vi "Index Tags.vi"(4 "Write?":bool, 6 "Data Type":T1, 8 "error in (no error)":errorcluster, 9 "Tag":string, 10 "Group Index":i32, 11 "bt_Blackboard in":refnum<class "Blackboard.lvclass">) -> (0 "error out":errorcluster, 1 "New Tag?":bool, 2 "Index":i32, 3 "bt_Blackboard out":refnum<class "Blackboard.lvclass">)   [LabVIEW 2021, in "Blackboard.lvclass"]
uses:
  Blackboard.lvclass
  Data Type.ctl
  Blackboard.lvclass/Blackboard.ctl
  Status Type.ctl
  <vilib>/Utility/error.llb/Error Cluster From Error Code.vi
  <vilib>/ErrorRing/Error Ring.xnode
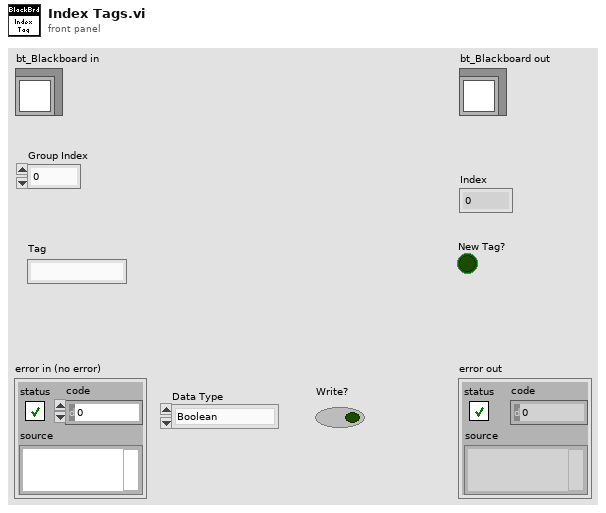
[diagram p1: front panel]
types:
  T1 = typedef "Blackboard.lvclass/Data Type.ctl" = enum16{"Boolean", "String", "DBL", "SGL", "EXT", "U8", "U16", "U32", "U64", "I8", "I16", "I32", "I64", "CDBL", "CSGL", "CEXT", "Time", "Variant", "Waveform"}
  T2 = typedef "Blackboard.lvclass/Status Type.ctl" = cluster{"Read?":u32, "Write?":u32, "Data Type":T1}
  T3 = typedef "Blackboard.lvclass/Data DVR Type.ctl" = cluster{"Tags":T4, "Status":refnum<data-value>, "Boolean":refnum<data-value>, "String":refnum<data-value>, "DBL":refnum<data-value>, "SGL":refnum<data-value>, "EXT":refnum<data-value>, "U8":refnum<data-value>, "U16":refnum<data-value>, "U32":refnum<data-value>, "U64":refnum<data-value>, "I8":refnum<data-value>, "I16":refnum<data-value>, "I32":refnum<data-value>, "I64":refnum<data-value>, "CDBL":refnum<data-value>, "CSGL":refnum<data-value>, "CEXT":refnum<data-value>, "Time":refnum<data-value>, "Variant":refnum<data-value>, "Waveform":refnum<data-value>}
  T4 = typedef "Blackboard.lvclass/Tags Map Type.ctl" = map{string, cluster{"Data Index":i32, "Status Index":i32}}
  T5 = typedef "Blackboard.lvclass/Group Map Type.ctl" = map{string, i32}
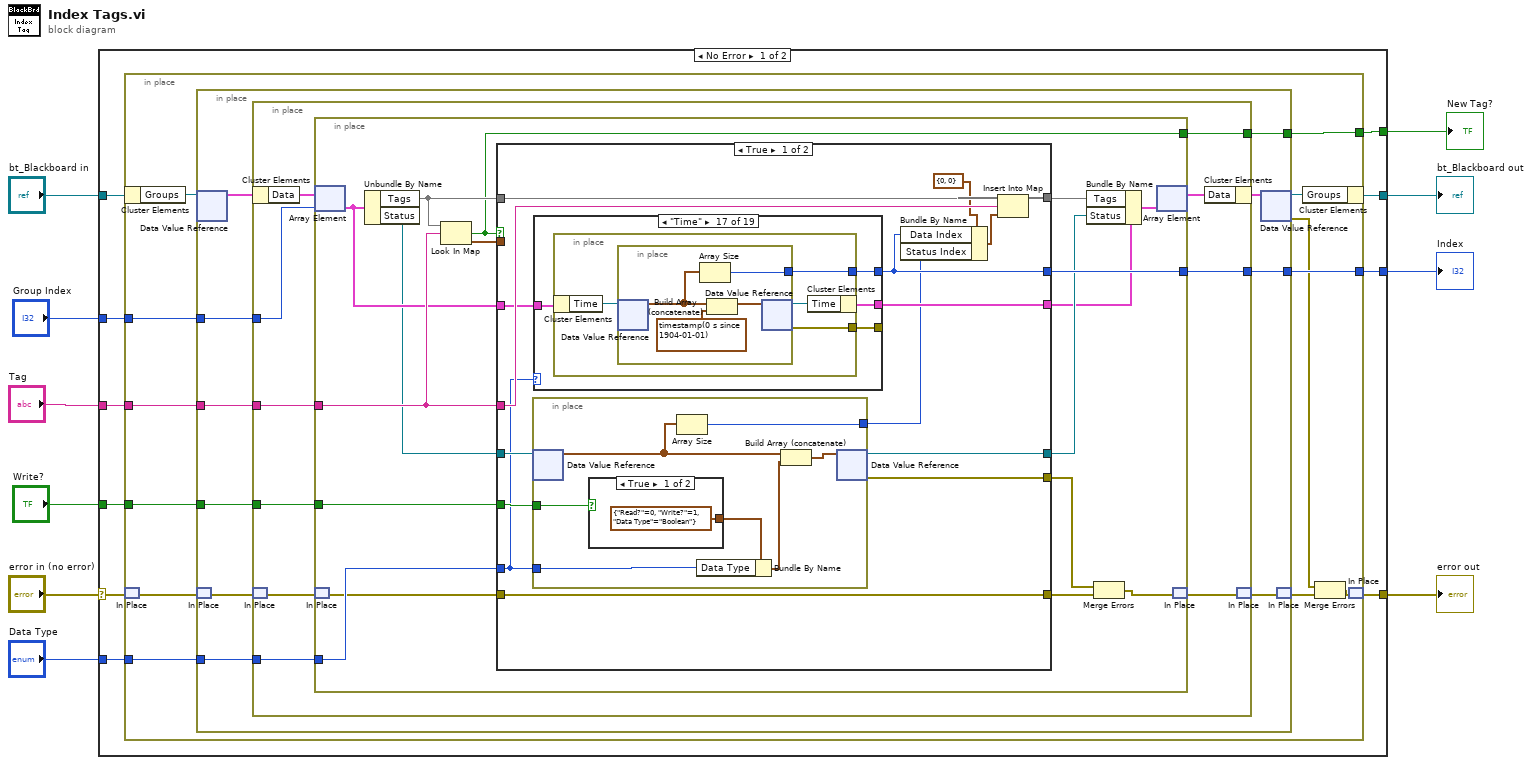
[diagram p0: block diagram]
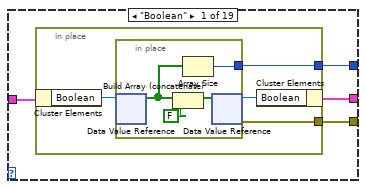
[diagram p2: hidden frame]
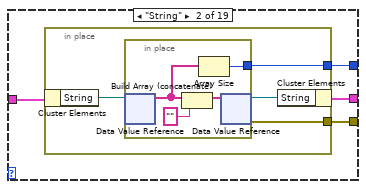
[diagram p3: hidden frame]
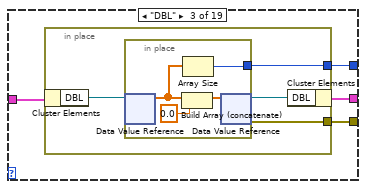
[diagram p4: hidden frame]
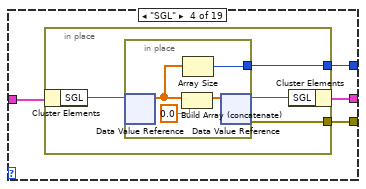
[diagram p5: hidden frame]
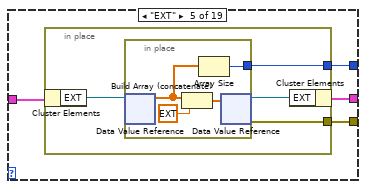
[diagram p6: hidden frame]
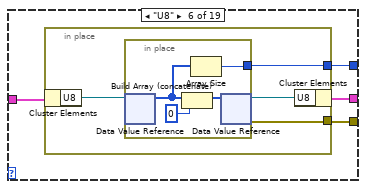
[diagram p7: hidden frame]
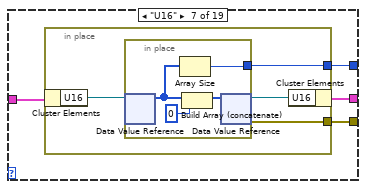
[diagram p8: hidden frame]
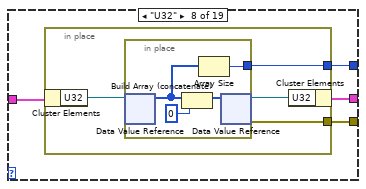
[diagram p9: hidden frame]
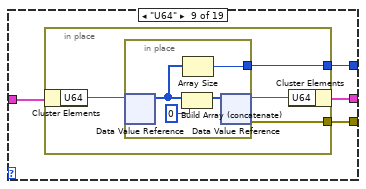
[diagram p10: hidden frame]
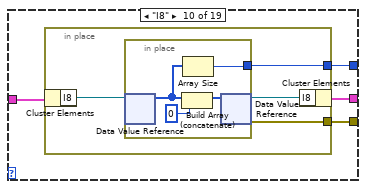
[diagram p11: hidden frame]
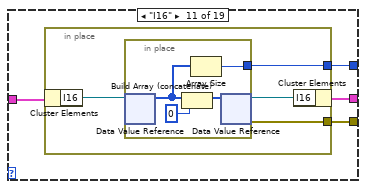
[diagram p12: hidden frame]
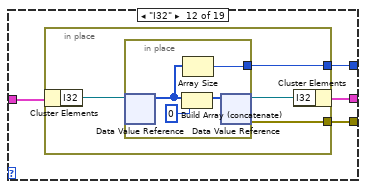
[diagram p13: hidden frame]
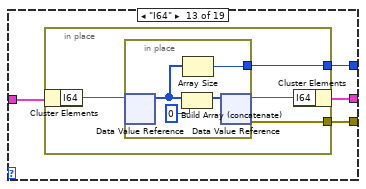
[diagram p14: hidden frame]
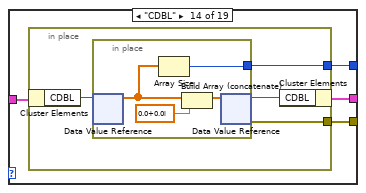
[diagram p15: hidden frame]
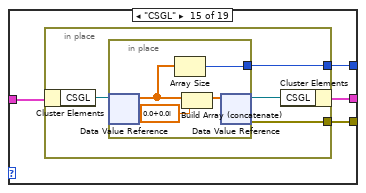
[diagram p16: hidden frame]
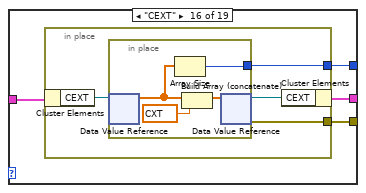
[diagram p17: hidden frame]
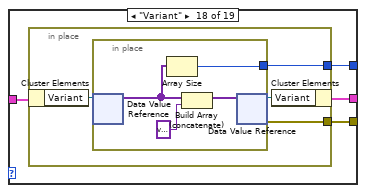
[diagram p18: hidden frame]
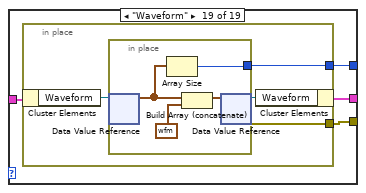
[diagram p19: hidden frame]
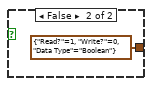
[diagram p20: hidden frame]
diagram:
  n1 = case shown="No Error" "error in (no error)" {
    selector: "error in (no error)" -> [w13 w366]
    tunnel: [w12 w366] -> w9
    tunnel: [w17 w365] -> w7
    tunnel: "bt_Blackboard in" -> [w18 w365]
    tunnel: "Tag" -> [w20 _]
    tunnel: [w19 _] -> w5
    tunnel: "Group Index" -> [w16 _]
    tunnel: "Write?" -> [w15 _]
    tunnel: "Data Type" -> [w14 _]
    tunnel: [w11 _] -> w1
    frame No Error {
      n2 = in-place {
        in-place-border: w20 -> [w32]
        in-place-border: [w31] -> w19
        in-place-border: w16 -> [w30]
        in-place-border: w15 -> [w29]
        in-place-border: w14 -> [w28]
        in-place-border: [w27] -> w11
        n3 = in-place-cluster #1(w18) -> ("Groups"=w26:refnum<data-value>)
        n4 = in-place-match #2(w13) -> (w25:errorcluster)
        n5 = in-place {
          in-place-border: w32 -> [w42]
          in-place-border: [w41] -> w31
          in-place-border: w30 -> [w40]
          in-place-border: w29 -> [w39]
          in-place-border: w28 -> [w38]
          in-place-border: [w37] -> w27
          n6 = in-place-dvr #3(w26) -> (w36:cluster{"Data":T3[], "Map":T5, "Status":u32[]})  [unwired: 1 out]
          n7 = in-place-match #4(w25) -> (w34:errorcluster)
          n8 = in-place {
            in-place-border: w42 -> [w52]
            in-place-border: [w51] -> w41
            in-place-border: w40 -> [w50]
            in-place-border: w39 -> [w49]
            in-place-border: w38 -> [w48]
            in-place-border: [w47] -> w37
            n9 = in-place-cluster #5(w36) -> ("Data"=w46:T3[])
            n10 = in-place-match #6(w34) -> (w44:errorcluster)
            n11 = in-place {
              in-place-border: w52 -> [w69]
              in-place-border: [w63] -> w51
              in-place-border: w49 -> [w68]
              in-place-border: w48 -> [w66]
              in-place-border: [w53] -> w47
              n12 = in-place-array #7(w46, w50) -> (w62:T3)
              n13 = in-place-match #8(w44) -> (w65:errorcluster)
              n14 = Unbundle By Name(w62) -> ("Tags"=w60:T4, "Status"=w57:refnum<data-value>)
              n15 = Look In Map(map=w60, key=w69) -> (key not found?=w53:bool, value=w58:cluster{"Data Index":i32, "Status Index":i32})  [unwired: 1 in]
              n16 = case shown="True" w53 {
                tunnel: w60 -> [w79 w327]
                tunnel: [w78 w327] -> w59
                tunnel: w69 -> [w77 _]
                tunnel: [w81 w324] -> w56
                tunnel: w68 -> [w84 w333]
                tunnel: w66 -> [w74 w332]
                tunnel: w65 -> [w83 w331]
                tunnel: [w83 w330] -> w61
                tunnel: w58 -> [_ w329]
                tunnel: [w73 w328] -> w63
                tunnel: w57 -> [w82 w325]
                tunnel: [w80 w323] -> w55
                tunnel: w62 -> [w76 w322]
                tunnel: [w75 w322] -> w54
                frame True {
                  n17 = in-place {
                    in-place-border: w84 -> [w319]
                    in-place-border: w74 -> [w315]
                    in-place-border: [w313] -> w70
                    n18 = in-place-dvr #9(w82) -> (w314:T2[])  [unwired: 1 out]
                    n19 = case shown="True" w319 {
                      tunnel: [T2 {"Read?"=0, "Write?"=1, "Data Type"=enum."Boolean"} ("Status") T2 {"Read?"=1, "Write?"=0, "Data Type"=enum."Boolean"} ("Status")] -> w318
                      frame True {
                      }
                      frame False {
                      }
                    }
                    n20 = Array Size(array=w314) -> (size(s)=w313:i32)
                    n21 = Bundle By Name(cluster=w318, "Data Type"=w315) -> (w316:T2)
                    n22 = Build Array (concatenate)(w314, w316) -> (w317:T2[])
                    n23 = in-place-dvr #9(w317) -> (w81:refnum<data-value>, w80:errorcluster)
                  }
                  n24 = case shown="\"Time\"" w74 {
                    tunnel: w76 -> [w88 w100 w112 w124 w136 w148 w160 w172 w184 w196 w208 w220 w232 w244 w256 w268 w280 w292 w304]
                    tunnel: [w87 w99 w111 w123 w135 w147 w159 w171 w183 w195 w207 w219 w231 w243 w255 w267 w279 w291 w303] -> w75
                    tunnel: [w86 w98 w110 w122 w134 w146 w158 w170 w182 w194 w206 w218 w230 w242 w254 w266 w278 w290 w302] -> _
                    tunnel: [w85 w97 w109 w121 w133 w145 w157 w169 w181 w193 w205 w217 w229 w241 w253 w265 w277 w289 w301] -> w73
                    frame "Boolean" {
                      n25 = in-place {
                        in-place-border: [w90] -> w86
                        in-place-border: [w89] -> w85
                        n26 = in-place-cluster #10(w88) -> ("Boolean"=w92:refnum<data-value>)
                        n27 = in-place {
                          in-place-border: [w93] -> w89
                          n28 = in-place-dvr #11(w92) -> (w94:bool[])  [unwired: 1 out]
                          n29 = Build Array (concatenate)(w94, FALSE) -> (w96:bool[])
                          n30 = Array Size(array=w94) -> (size(s)=w93:i32)
                          n31 = in-place-dvr #11(w96) -> (w91:refnum<data-value>, w90:errorcluster)
                        }
                        n32 = in-place-cluster #10("Boolean"=w91) -> (w87:T3)
                      }
                    }
                    frame "String" {
                      n33 = in-place {
                        in-place-border: [w102] -> w98
                        in-place-border: [w101] -> w97
                        n34 = in-place-cluster #12(w100) -> ("String"=w104:refnum<data-value>)
                        n35 = in-place {
                          in-place-border: [w105] -> w101
                          n36 = in-place-dvr #13(w104) -> (w106:string[])  [unwired: 1 out]
                          n37 = Build Array (concatenate)(w106, "") -> (w108:string[])
                          n38 = Array Size(array=w106) -> (size(s)=w105:i32)
                          n39 = in-place-dvr #13(w108) -> (w103:refnum<data-value>, w102:errorcluster)
                        }
                        n40 = in-place-cluster #12("String"=w103) -> (w99:T3)
                      }
                    }
                    frame "DBL" {
                      n41 = in-place {
                        in-place-border: [w114] -> w110
                        in-place-border: [w113] -> w109
                        n42 = in-place-cluster #14(w112) -> ("DBL"=w116:refnum<data-value>)
                        n43 = in-place {
                          in-place-border: [w117] -> w113
                          n44 = in-place-dvr #15(w116) -> (w118:dbl[])  [unwired: 1 out]
                          n45 = Build Array (concatenate)(w118, 0.0) -> (w120:dbl[])
                          n46 = Array Size(array=w118) -> (size(s)=w117:i32)
                          n47 = in-place-dvr #15(w120) -> (w115:refnum<data-value>, w114:errorcluster)
                        }
                        n48 = in-place-cluster #14("DBL"=w115) -> (w111:T3)
                      }
                    }
                    frame "SGL" {
                      n49 = in-place {
                        in-place-border: [w126] -> w122
                        in-place-border: [w125] -> w121
                        n50 = in-place-cluster #16(w124) -> ("SGL"=w128:refnum<data-value>)
                        n51 = in-place {
                          in-place-border: [w129] -> w125
                          n52 = in-place-dvr #17(w128) -> (w130:sgl[])  [unwired: 1 out]
                          n53 = Build Array (concatenate)(w130, sgl 0.0) -> (w132:sgl[])
                          n54 = Array Size(array=w130) -> (size(s)=w129:i32)
                          n55 = in-place-dvr #17(w132) -> (w127:refnum<data-value>, w126:errorcluster)
                        }
                        n56 = in-place-cluster #16("SGL"=w127) -> (w123:T3)
                      }
                    }
                    frame "EXT" {
                      n57 = in-place {
                        in-place-border: [w138] -> w134
                        in-place-border: [w137] -> w133
                        n58 = in-place-cluster #18(w136) -> ("EXT"=w140:refnum<data-value>)
                        n59 = in-place {
                          in-place-border: [w141] -> w137
                          n60 = in-place-dvr #19(w140) -> (w142:ext[])  [unwired: 1 out]
                          n61 = Build Array (concatenate)(w142, ext 0.0) -> (w143:ext[])
                          n62 = Array Size(array=w142) -> (size(s)=w141:i32)
                          n63 = in-place-dvr #19(w143) -> (w139:refnum<data-value>, w138:errorcluster)
                        }
                        n64 = in-place-cluster #18("EXT"=w139) -> (w135:T3)
                      }
                    }
                    frame "U8" {
                      n65 = in-place {
                        in-place-border: [w150] -> w146
                        in-place-border: [w149] -> w145
                        n66 = in-place-cluster #20(w148) -> ("U8"=w152:refnum<data-value>)
                        n67 = in-place {
                          in-place-border: [w153] -> w149
                          n68 = in-place-dvr #21(w152) -> (w154:u8[])  [unwired: 1 out]
                          n69 = Build Array (concatenate)(w154, u8 0) -> (w156:u8[])
                          n70 = Array Size(array=w154) -> (size(s)=w153:i32)
                          n71 = in-place-dvr #21(w156) -> (w151:refnum<data-value>, w150:errorcluster)
                        }
                        n72 = in-place-cluster #20("U8"=w151) -> (w147:T3)
                      }
                    }
                    frame "U16" {
                      n73 = in-place {
                        in-place-border: [w162] -> w158
                        in-place-border: [w161] -> w157
                        n74 = in-place-cluster #22(w160) -> ("U16"=w164:refnum<data-value>)
                        n75 = in-place {
                          in-place-border: [w165] -> w161
                          n76 = in-place-dvr #23(w164) -> (w166:u16[])  [unwired: 1 out]
                          n77 = Array Size(array=w166) -> (size(s)=w165:i32)
                          n78 = Build Array (concatenate)(w166, u16 0) -> (w168:u16[])
                          n79 = in-place-dvr #23(w168) -> (w163:refnum<data-value>, w162:errorcluster)
                        }
                        n80 = in-place-cluster #22("U16"=w163) -> (w159:T3)
                      }
                    }
                    frame "U32" {
                      n81 = in-place {
                        in-place-border: [w174] -> w170
                        in-place-border: [w173] -> w169
                        n82 = in-place-cluster #24(w172) -> ("U32"=w176:refnum<data-value>)
                        n83 = in-place {
                          in-place-border: [w177] -> w173
                          n84 = in-place-dvr #25(w176) -> (w178:u32[])  [unwired: 1 out]
                          n85 = Build Array (concatenate)(w178, u32 0) -> (w180:u32[])
                          n86 = Array Size(array=w178) -> (size(s)=w177:i32)
                          n87 = in-place-dvr #25(w180) -> (w175:refnum<data-value>, w174:errorcluster)
                        }
                        n88 = in-place-cluster #24("U32"=w175) -> (w171:T3)
                      }
                    }
                    frame "U64" {
                      n89 = in-place {
                        in-place-border: [w186] -> w182
                        in-place-border: [w185] -> w181
                        n90 = in-place-cluster #26(w184) -> ("U64"=w188:refnum<data-value>)
                        n91 = in-place {
                          in-place-border: [w189] -> w185
                          n92 = in-place-dvr #27(w188) -> (w190:u64[])  [unwired: 1 out]
                          n93 = Build Array (concatenate)(w190, u64 0) -> (w192:u64[])
                          n94 = Array Size(array=w190) -> (size(s)=w189:i32)
                          n95 = in-place-dvr #27(w192) -> (w187:refnum<data-value>, w186:errorcluster)
                        }
                        n96 = in-place-cluster #26("U64"=w187) -> (w183:T3)
                      }
                    }
                    frame "I8" {
                      n97 = in-place {
                        in-place-border: [w198] -> w194
                        in-place-border: [w197] -> w193
                        n98 = in-place-cluster #28(w196) -> ("I8"=w200:refnum<data-value>)
                        n99 = in-place {
                          in-place-border: [w201] -> w197
                          n100 = in-place-dvr #29(w200) -> (w202:i8[])  [unwired: 1 out]
                          n101 = Build Array (concatenate)(w202, i8 0) -> (w204:i8[])
                          n102 = Array Size(array=w202) -> (size(s)=w201:i32)
                          n103 = in-place-dvr #29(w204) -> (w199:refnum<data-value>, w198:errorcluster)
                        }
                        n104 = in-place-cluster #28("I8"=w199) -> (w195:T3)
                      }
                    }
                    frame "I16" {
                      n105 = in-place {
                        in-place-border: [w210] -> w206
                        in-place-border: [w209] -> w205
                        n106 = in-place-cluster #30(w208) -> ("I16"=w212:refnum<data-value>)
                        n107 = in-place {
                          in-place-border: [w213] -> w209
                          n108 = in-place-dvr #31(w212) -> (w214:i16[])  [unwired: 1 out]
                          n109 = Build Array (concatenate)(w214, i16 0) -> (w216:i16[])
                          n110 = Array Size(array=w214) -> (size(s)=w213:i32)
                          n111 = in-place-dvr #31(w216) -> (w211:refnum<data-value>, w210:errorcluster)
                        }
                        n112 = in-place-cluster #30("I16"=w211) -> (w207:T3)
                      }
                    }
                    frame "I32" {
                      n113 = in-place {
                        in-place-border: [w222] -> w218
                        in-place-border: [w221] -> w217
                        n114 = in-place-cluster #32(w220) -> ("I32"=w224:refnum<data-value>)
                        n115 = in-place {
                          in-place-border: [w225] -> w221
                          n116 = in-place-dvr #33(w224) -> (w226:i32[])  [unwired: 1 out]
                          n117 = Build Array (concatenate)(w226, 0) -> (w228:i32[])
                          n118 = Array Size(array=w226) -> (size(s)=w225:i32)
                          n119 = in-place-dvr #33(w228) -> (w223:refnum<data-value>, w222:errorcluster)
                        }
                        n120 = in-place-cluster #32("I32"=w223) -> (w219:T3)
                      }
                    }
                    frame "I64" {
                      n121 = in-place {
                        in-place-border: [w234] -> w230
                        in-place-border: [w233] -> w229
                        n122 = in-place-cluster #34(w232) -> ("I64"=w236:refnum<data-value>)
                        n123 = in-place {
                          in-place-border: [w237] -> w233
                          n124 = in-place-dvr #35(w236) -> (w238:i64[])  [unwired: 1 out]
                          n125 = Build Array (concatenate)(w238, i64 0) -> (w240:i64[])
                          n126 = Array Size(array=w238) -> (size(s)=w237:i32)
                          n127 = in-place-dvr #35(w240) -> (w235:refnum<data-value>, w234:errorcluster)
                        }
                        n128 = in-place-cluster #34("I64"=w235) -> (w231:T3)
                      }
                    }
                    frame "CDBL" {
                      n129 = in-place {
                        in-place-border: [w246] -> w242
                        in-place-border: [w245] -> w241
                        n130 = in-place-cluster #36(w244) -> ("CDBL"=w248:refnum<data-value>)
                        n131 = in-place {
                          in-place-border: [w249] -> w245
                          n132 = in-place-dvr #37(w248) -> (w250:cdb[])  [unwired: 1 out]
                          n133 = Array Size(array=w250) -> (size(s)=w249:i32)
                          n134 = Build Array (concatenate)(w250, cdb 0.0+0.0i) -> (w252:cdb[])
                          n135 = in-place-dvr #37(w252) -> (w247:refnum<data-value>, w246:errorcluster)
                        }
                        n136 = in-place-cluster #36("CDBL"=w247) -> (w243:T3)
                      }
                    }
                    frame "CSGL" {
                      n137 = in-place {
                        in-place-border: [w258] -> w254
                        in-place-border: [w257] -> w253
                        n138 = in-place-cluster #38(w256) -> ("CSGL"=w260:refnum<data-value>)
                        n139 = in-place {
                          in-place-border: [w261] -> w257
                          n140 = in-place-dvr #39(w260) -> (w262:csg[])  [unwired: 1 out]
                          n141 = Array Size(array=w262) -> (size(s)=w261:i32)
                          n142 = Build Array (concatenate)(w262, csg 0.0+0.0i) -> (w264:csg[])
                          n143 = in-place-dvr #39(w264) -> (w259:refnum<data-value>, w258:errorcluster)
                        }
                        n144 = in-place-cluster #38("CSGL"=w259) -> (w255:T3)
                      }
                    }
                    frame "CEXT" {
                      n145 = in-place {
                        in-place-border: [w270] -> w266
                        in-place-border: [w269] -> w265
                        n146 = in-place-cluster #40(w268) -> ("CEXT"=w272:refnum<data-value>)
                        n147 = in-place {
                          in-place-border: [w273] -> w269
                          n148 = in-place-dvr #41(w272) -> (w274:cxt[])  [unwired: 1 out]
                          n149 = Array Size(array=w274) -> (size(s)=w273:i32)
                          n150 = Build Array (concatenate)(w274, cxt 0.0+0.0i) -> (w276:cxt[])
                          n151 = in-place-dvr #41(w276) -> (w271:refnum<data-value>, w270:errorcluster)
                        }
                        n152 = in-place-cluster #40("CEXT"=w271) -> (w267:T3)
                      }
                    }
                    frame "Time" {
                      n153 = in-place {
                        in-place-border: [w282] -> w278
                        in-place-border: [w281] -> w277
                        n154 = in-place-cluster #42(w280) -> ("Time"=w284:refnum<data-value>)
                        n155 = in-place {
                          in-place-border: [w285] -> w281
                          n156 = in-place-dvr #43(w284) -> (w286:timestamp[])  [unwired: 1 out]
                          n157 = Array Size(array=w286) -> (size(s)=w285:i32)
                          n158 = Build Array (concatenate)(w286, timestamp(0 s since 1904-01-01)) -> (w288:timestamp[])
                          n159 = in-place-dvr #43(w288) -> (w283:refnum<data-value>, w282:errorcluster)
                        }
                        n160 = in-place-cluster #42("Time"=w283) -> (w279:T3)
                      }
                    }
                    frame "Variant" {
                      n161 = in-place {
                        in-place-border: [w294] -> w290
                        in-place-border: [w293] -> w289
                        n162 = in-place-cluster #44(w292) -> ("Variant"=w296:refnum<data-value>)
                        n163 = in-place {
                          in-place-border: [w297] -> w293
                          n164 = in-place-dvr #45(w296) -> (w298:variant[])  [unwired: 1 out]
                          n165 = Array Size(array=w298) -> (size(s)=w297:i32)
                          n166 = Build Array (concatenate)(w298, variant) -> (w300:variant[])
                          n167 = in-place-dvr #45(w300) -> (w295:refnum<data-value>, w294:errorcluster)
                        }
                        n168 = in-place-cluster #44("Variant"=w295) -> (w291:T3)
                      }
                    }
                    frame "Waveform" {
                      n169 = in-place {
                        in-place-border: [w306] -> w302
                        in-place-border: [w305] -> w301
                        n170 = in-place-cluster #46(w304) -> ("Waveform"=w308:refnum<data-value>)
                        n171 = in-place {
                          in-place-border: [w309] -> w305
                          n172 = in-place-dvr #47(w308) -> (w310:waveform(dbl)[])  [unwired: 1 out]
                          n173 = Array Size(array=w310) -> (size(s)=w309:i32)
                          n174 = Build Array (concatenate)(w310, waveform(dbl) {"t0"=timestamp(0 s since 1904-01-01), "dt"=1.0, "Y"=[]} ("Waveform")) -> (w312:waveform(dbl)[])
                          n175 = in-place-dvr #47(w312) -> (w307:refnum<data-value>, w306:errorcluster)
                        }
                        n176 = in-place-cluster #46("Waveform"=w307) -> (w303:T3)
                      }
                    }
                  }
                  n177 = Bundle By Name(cluster=cluster{"Data Index":i32, "Status Index":i32} {"Data Index"=0, "Status Index"=0} ("value"), "Data Index"=w73, "Status Index"=w70) -> (w71:cluster{"Data Index":i32, "Status Index":i32})
                  n178 = Insert Into Map(map in=w79, key=w77, value=w71) -> (map out=w78:T4)  [unwired: 2 out]
                }
                frame False {
                  (unwired) FALSE
                  n179 = Unbundle By Name(w329) -> ("Data Index"=w328:i32, "Status Index"=w326:i32)
                  n180 = in-place {
                    in-place-border: w333 -> [w340]
                    in-place-border: w332 -> [w339]
                    in-place-border: w331 -> [w338]
                    in-place-border: [w337] -> w330
                    in-place-border: w326 -> [w336]
                    n181 = in-place-dvr #48(w325) -> (w335:T2[])  [unwired: 1 out]
                    n182 = in-place {
                      in-place-border: w340 -> [w349]
                      in-place-border: w339 -> [w346]
                      in-place-border: w338 -> [w343]
                      in-place-border: [w342] -> w337
                      n183 = in-place-array #49(w335, w336) -> (w347:T2)
                      n184 = xnode "Error Ring"() -> ("error out"=w341:errorcluster)
                      n185 = case shown="True" w349 {
                        tunnel: w347 -> [w358 w362]
                        tunnel: [w357 w361] -> w348
                        frame True {
                          n186 = in-place {
                            n187 = in-place-cluster #50(w358) -> ("Write?"=w360:u32)
                            n188 = Increment(x=w360) -> (x+1=w359:u32)
                            n189 = in-place-cluster #50("Write?"=w359) -> (w357:T2)
                          }
                        }
                        frame False {
                          n190 = in-place {
                            n191 = in-place-cluster #51(w362) -> ("Read?"=w364:u32)
                            n192 = Increment(x=w364) -> (x+1=w363:u32)
                            n193 = in-place-cluster #51("Read?"=w363) -> (w361:T2)
                          }
                        }
                      }
                      n194 = Unbundle By Name(w347) -> ("Data Type"=w345:T1)
                      n195 = Not Equal?(x=w345, y=w346) -> (x != y?=w344:bool)
                      n196 = case shown="True" w344 {
                        tunnel: w343 -> [w355 _]
                        tunnel: [w355 w356] -> w342
                        tunnel: w341 -> [_ w356]
                        frame False {
                        }
                        frame True {
                        }
                      }
                      n197 = in-place-array #49(w348) -> (w334:T2[])  [unwired: 1 out]
                    }
                    n198 = in-place-dvr #48(w334) -> (w324:refnum<data-value>, w323:errorcluster)
                  }
                }
              }
              n199 = Bundle By Name(cluster=w54, "Tags"=w59, "Status"=w56) -> (w67:T3)
              n200 = Merge Errors(w55, w61) -> (w64:errorcluster)
              n201 = in-place-array #7(w67) -> (w45:T3[])  [unwired: 1 out]
              n202 = in-place-match #8(w64) -> (w43:errorcluster)
            }
            n203 = in-place-cluster #5("Data"=w45) -> (w35:cluster{"Data":T3[], "Map":T5, "Status":u32[]})
            n204 = in-place-match #6(w43) -> (w33:errorcluster)
          }
          n205 = in-place-dvr #3(w35) -> (w23:refnum<data-value>, w21:errorcluster)
          n206 = in-place-match #4(w33) -> (w24:errorcluster)
        }
        n207 = in-place-cluster #1("Groups"=w23) -> (w17:refnum<class "Blackboard.lvclass">)
        n208 = Merge Errors(w21, w24) -> (w22:errorcluster)
        n209 = in-place-match #2(w22) -> (w12:errorcluster)
      }
    }
    frame Error {
    }
  }
  "error out" <- w9
  "bt_Blackboard out" <- w7
  "Index" <- w5
  "New Tag?" <- w1
